vi "Read Process Kill timeout.vi"(11 "SMO in":refnum<class "SMO.lvclass">) -> (2 "Process Kill timeout (ms)":i32=500, 3 "SMO out":refnum<class "SMO.lvclass">)   [LabVIEW 2021, in "smo.lvlib" / "SMO.lvclass"]
uses:
  SMO.lvclass
  SMO.lvclass/SMO.ctl
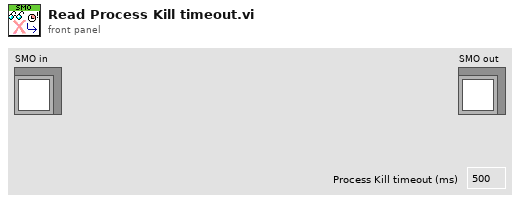
[diagram p1: front panel]
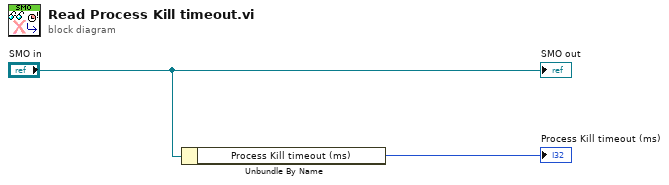
[diagram p0: block diagram]
diagram:
  n1 = Unbundle By Name("SMO in") -> ("Process Kill timeout (ms)"=→"Process Kill timeout (ms)":i32)
  "SMO out" <- "SMO in"
